vi "Init Msg.vi"(10 "Msg Input":refnum<class "Msg Input.lvclass">) -> (2 "Msg":refnum<class "Msg.lvclass">)   [LabVIEW 2020, in "jettl.lvlib" / "Stopping jettl Msg.lvlib" / "Stopping Msg.lvlib"]
doc: "jettl 6.12.1.94\nNathan Davis - Nathan Davis\nCopyright (c) 2026, Nathan Davis\nMIT"
uses:
  Stopping Msg.lvlib
  Msg/Msg.lvclass
  Msg Input/Msg Input.lvclass
  Stopping Msg/Stopping Msg.lvclass
  C:/git/jettl/src/jettl/jettl/Msg/Msg.lvclass
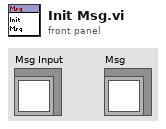
[diagram p1: front panel]
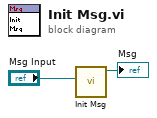
[diagram p0: block diagram]
diagram:
  n1 = call "Init Msg.vi"("Msg Input"="Msg Input") -> ("Stopping Msg out"=→"Msg":refnum<class "Stopping Msg.lvclass">)  [unwired: 10 in]
